vi "Get Configuration File Target Path.vi"(8 "error in (no error)":errorcluster, 11 "Item Ref in":T1 format="%.0x") -> (0 "error out":errorcluster, 2 "configuration target path":path, 3 "Item Ref out":T1 format="%.0x")   [LabVIEW 2021, in "DSF Shared.lvlib"]
uses:
  DSF Shared.lvlib
  <vilib>/NI VeriStand/Custom Device API/Custom Device Item Ref.ctl
  <vilib>/NI VeriStand/Custom Device API/Get Item Property (Path).vi
  <vilib>/NI VeriStand/Custom Device API/Custom Device API.lvlib
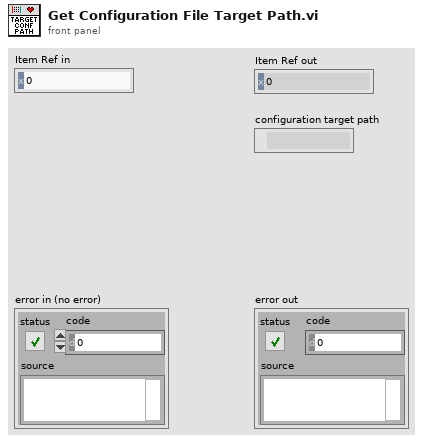
[diagram p1: front panel]
types:
  T1 = typedef "Custom Device API.lvlib/Custom Device Item Ref.ctl" = u64
  T2 = typedef "Custom Device API.lvlib/Custom Device Target Type.ctl" = enum16{"PharLap", "VxWorks", "Windows", "Linux_32_ARM", "Linux_x64"}
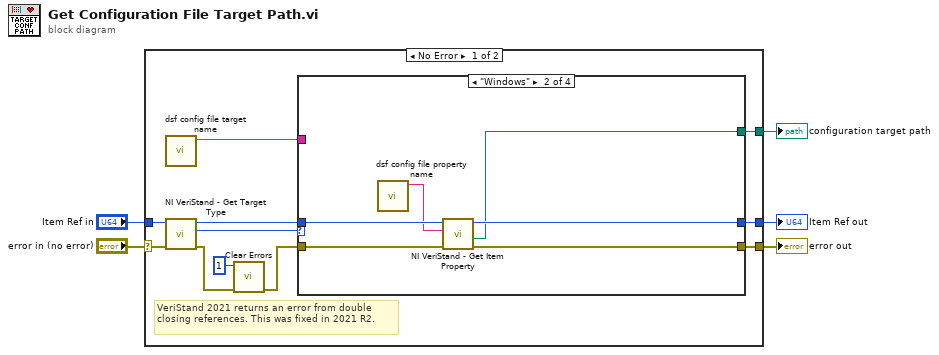
[diagram p0: block diagram]
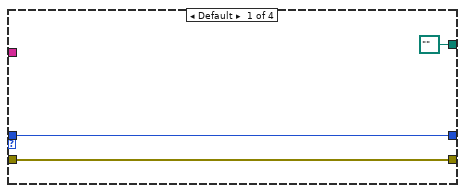
[diagram p2: hidden frame]
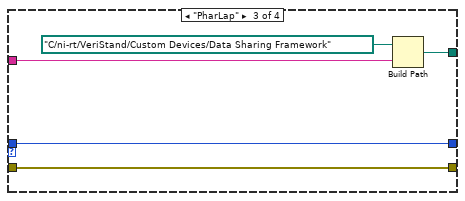
[diagram p3: hidden frame]
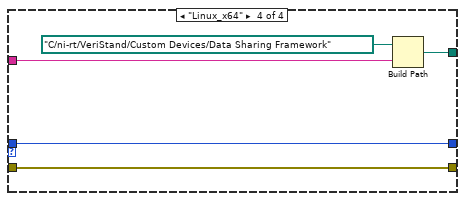
[diagram p4: hidden frame]
diagram:
  n1 = case shown="No Error" "error in (no error)" {
    selector: "error in (no error)" -> [w16 w36]
    tunnel: "Item Ref in" -> [w15 w37]
    tunnel: [w11 _] -> w3
    tunnel: [w10 w36] -> w2
    tunnel: [w9 w37] -> w1
    frame No Error {
      # "VeriStand 2021 returns an error from double closing references. This was fixed in 2021 R2."
      n2 = call "dsf config file target name.vi"() -> ("config file target name"=w8:string)  [unwired: 11 in]
      n3 = call <vilib>:"NI VeriStand - Get Target Type.vi"("error in (no error)"=w16, "Item Ref in"=w15) -> ("error out"=w12:errorcluster, "Target Type"=w14:T2, "Item Ref out"=w13:T1)  [unwired: 7 in]
      n4 = call <vilib>:"Clear Errors.vi"("error in (no error)"=w12, "specific error code to clear (0: all)"=1) -> ("error out"=w7:errorcluster)  [unwired: 4 in, 1 out]
      n5 = case shown="\"Windows\"" w14 {
        tunnel: w13 -> [w19 w25 w26 w31]
        tunnel: w7 -> [w18 w24 w27 w32]
        tunnel: w8 -> [_ _ w29 w34]
        tunnel: [path "" ("appended path") w21 w28 w33] -> w11
        tunnel: [w18 w22 w27 w32] -> w10
        tunnel: [w19 w23 w26 w31] -> w9
        frame Default {
        }
        frame "Windows" {
          n6 = call "dsf config file property name.vi"() -> ("file path property name"=w20:string)  [unwired: 11 in]
          n7 = call-poly <vilib>:"NI VeriStand - Get Item Property.vi"("error in (no error)"=w24, "Property Name"=w20, "Item Ref in"=w25) -> ("error out"=w22:errorcluster, "Value"=w21:path, "Item Ref out"=w23:T1)  [unwired: 5 in, 1 out]
        }
        frame "PharLap" {
          n8 = Build Path(base path=path "C:/ni-rt/VeriStand/Custom Devices/Data Sharing Framework" ("RT Destination"), name or relative path=w29) -> (appended path=w28:path)
        }
        frame "Linux_x64" {
          n9 = Build Path(base path=path "C:/ni-rt/VeriStand/Custom Devices/Data Sharing Framework" ("RT Destination"), name or relative path=w34) -> (appended path=w33:path)
        }
      }
    }
    frame Error {
    }
  }
  "Item Ref out" <- w1
  "error out" <- w2
  "configuration target path" <- w3
